vi "Python.vi"(8 "error in (no error)":errorcluster, 11 "module path":path) -> (0 "error out":errorcluster, 3 "return value":bool)   [LabVIEW 2024]
doc: "SubVi odpowiedzialne za wywołanie funkcji w pythonie oraz zwrócenie wartości True lub False w zależności czy rozpoznano twarz"
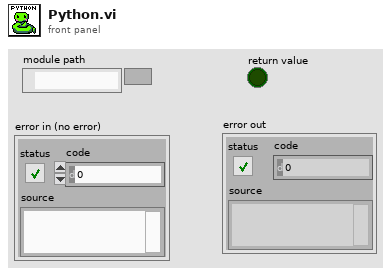
[diagram p1: front panel]
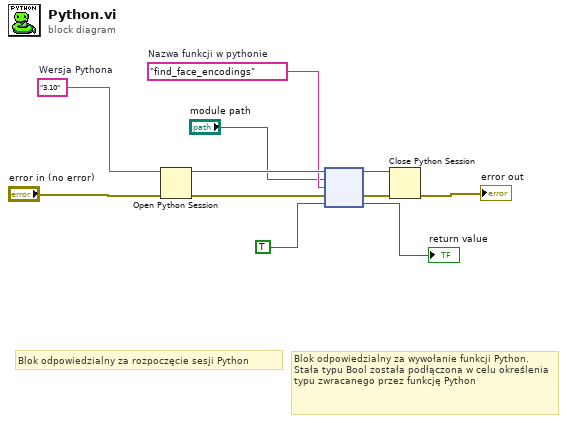
[diagram p0: block diagram]
diagram:
  w8 = "find_face_encodings"  # Nazwa funkcji w pythonie
  w11 = "3.10"  # Wersja Pythona
  # "Blok odpowiedzialny za wywołanie funkcji Python.\nStała typu Bool została podłączona w celu określenia typu zwracanego przez funkcję Python"
  # "Blok odpowiedzialny za rozpoczęcie sesji Python"
  n1 = Open Python Session(python version=w11, 3:"error in (no error)") -> (session out=w9:refnum<k35>, error out=w10:errorcluster)  [unwired: 1 in]
  n2 = node ("Python Node")(w9, "module path", w8, w10, TRUE) -> (w6:refnum<k35>, w5:errorcluster, →"return value":bool)  [unwired: 2 out]
  n3 = Close Python Session(session in=w6, error in=w5) -> (11:→"error out":errorcluster)
